vi "TurnForAngle.vi"() -> ()   [LabVIEW 2018]
uses:
  Framework/Robot Global Data.vi
panel:
  in  "NoWait":bool
  in  "Speed":dbl
  in  "Angle":dbl
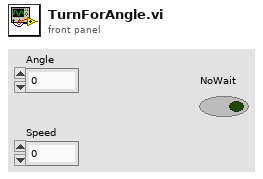
[diagram p1: front panel]
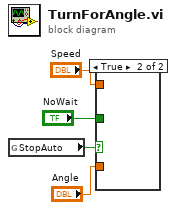
[diagram p0: block diagram]
diagram:
  n1 = global read "Robot Global Data.vi" "StopAuto"() -> (w2:bool)
  n2 = case shown="True" w2 {
    tunnel: "Angle" -> [_ _]
    tunnel: "Speed" -> [_ _]
    tunnel: "NoWait" -> [_ _]
    frame False {
    }
    frame True {
    }
  }
